vi "Camera.v5.vi"() -> ()   [LabVIEW 2015]
uses:
  Camera Properties.ctl
  Microscope Settings.ctl
  CameraState.ctl
  ModeEnum.ctl
  Stack_State.ctl
  Stack Track.ctl
  CameraControlTypeDef.ctl
  <vilib>/DAQmx/write.llb/DAQmx Write (Analog 1D Wfm NChan NSamp).vi
  <vilib>/DAQmx/create/channels.llb/DAQmx Create Channel (AO-Voltage-Basic).vi
  <vilib>/Waveform/WDTOps.llb/WDT Number of Waveform Samples DBL.vi
  <vilib>/DAQmx/configure/timing.llb/DAQmx Timing (Sample Clock).vi
  <vilib>/DAQmx/miscellaneous.llb/DAQmx Fill In Error Info.vi
  <vilib>/vision/NI_Vision_Development_Module.lvlib
  <vilib>/DAQmx/write.llb/DAQmx Write (Digital 1D Wfm NChan NSamp).vi
panel:
  out "Relax/ms":dbl
  in  "Tab Control":enum32{"Camera Settings", "Recording"}(tab)
  in  "Microscope Settings":T1={"Mode"=enum."XY", {"Scanning Mode"=12.0, "Slit Width /%"=5.0}, "Piezo Position /um"=0.0, "Exposure/ms"=40.0, "Samples per millisecond"=100.0, "Relax/ms"=10.0, "Readout Direction"=2.0, "Trigger Source"=2.0} {"Trigger Source" items=["Internal"=1.0, "External"=2.0]; "Readout Direction" items=["Forward"=1.0, "Backward"=2.0]; "?"."Scanning Mode" items=["Full Frame"=1.0, "Slit Scanning"=12.0]}
  in  "Scan":bool
  in  "Scan Continuously":bool
  out "error IO":errorcluster
  in  "V Height":dbl=2048.0 min=4.0 max=2048.0 step=4.0
  in  "V Offset":dbl min=0.0 max=0.0 step=4.0
  in  "H Offset":dbl min=0.0 max=0.0 step=4.0
  in  "H Width":dbl min=4.0 max=2048.0 step=4.0
  in  "Advanced DCAM Controls":i32(listbox) caption="Multicolumn Listbox"
  in  "Properties":T2=4211904 items=["SENSOR MODE"=4212128, "CCD MODE"=4212384, "READOUT MODE"=4211872, "ACTIVE VIEW INDEX"=4343136, "BITS PER CHANNEL"=4342976, "IMAGE PIXEL TYPE"=4343296, "BINNING"=4215968, "EXPOSURE TIME"=2049184, "CONTRAST GAIN"=3163312, "CONTRAST OFFSET"=3163328, "LIGHT MODE"=2114720, "SENSITIVITY"=2114992, "PHOTON IMAGING MODE"=2115200, "HIGH DYNAMIC RANGE MODE"=3163360, "WHITE BALANCE"=3163568, "TEMPERATURE"=2115232, "TEMPERATURE TARGET"=2115264, "SENSOR COOLER FAN"=2115296, "LINEBUNDLE HEIGHT"=4212192, "MECHANICAL SHUTTER"=2115488, "BACK FOCUS POSITION"=8422304, "TRIGGER CONNECTOR"=1066432, "TRIGGER SOURCE"=1066144, "OUTPUT TRIGGER SOURCE"=1852576, "TRIGGER GLOBAL EXPOSURE"=2049680, "FIRST TRIGGER BEHAVIOR"=2049696, "CHANNEL SYNC"=1852352, "READOUT DIRECTION"=4211904, "PRE HSYNC COUNT"=1852704, "INTERNAL LINE SPEED"=4191408, "INTERNAL LINE INVERVAL"=4191424]
  out "Waves":waveform(dbl)[](graph)
  out "Image":T3(plugin-control)
  out "Histogram":T4(graph)
  in  "stop":bool
  in  "Calibration":bool
  in  "MultiD Scan":bool
  in  "Stage Controller":bool
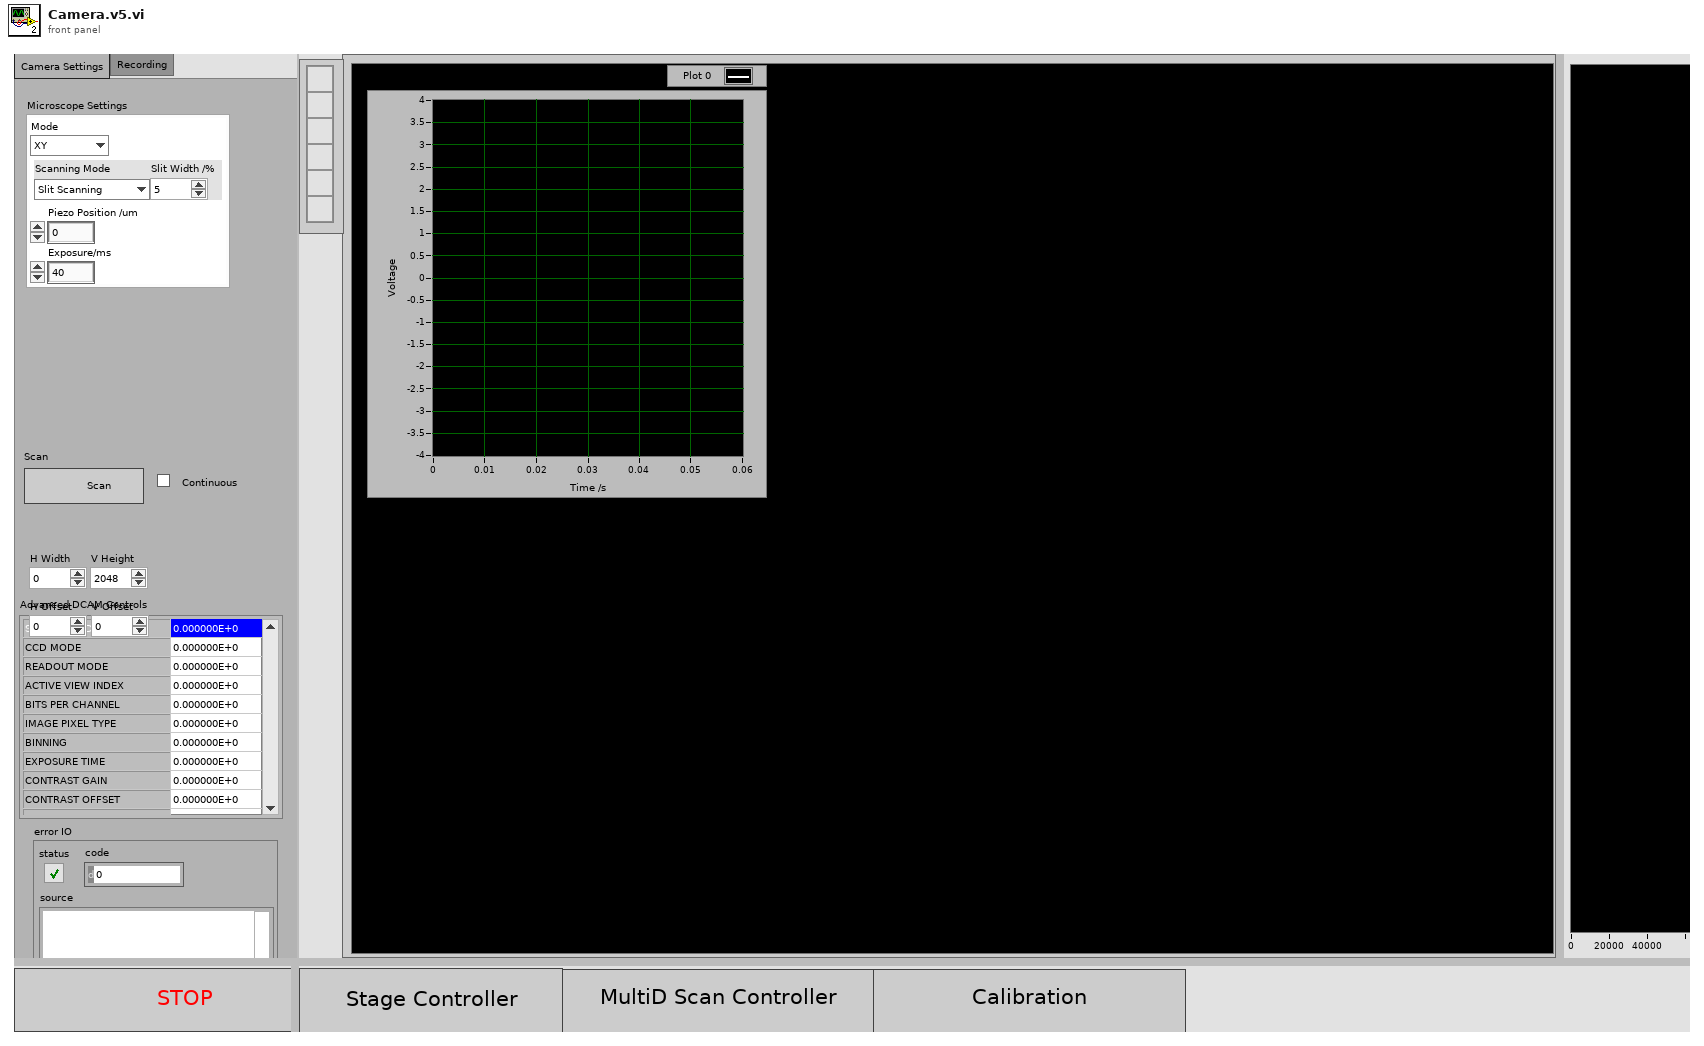
[diagram p1: front panel]
types:
  T1 = typedef "Microscope Settings.ctl" = cluster{"Mode":enum16{"X", "XY", "XYZ", "XYZT", "XYZC"}, cluster{"Scanning Mode":dbl, "Slit Width /%":dbl}, "Piezo Position /um":dbl, "Exposure/ms":dbl, "Samples per millisecond":dbl, "Relax/ms":dbl, "Readout Direction":dbl, "Trigger Source":dbl}
  T2 = typedef "Camera Properties.ctl" = u32
  T3 = typedef "IMAQ Image.ctl" = refnum<image>
  T4 = cluster{"Starting Value":sgl, "Incremental Value":sgl, "Histogram":u32[]}
  T5 = typedef "ModeEnum.ctl" = enum16{"Idle", "generateWaves", "runWaves", "stop"}
  T6 = cluster{"height":u32, "width":u32, "datatype":u32}
  T7 = typedef "CameraState.ctl" = enum16{"init", "active", "deinit"}
  T8 = typedef "CameraControlTypeDef.ctl" = enum16{"IntervalLineInt", "Ram Record", "HardDisk Record", "Disengage Update", "Update", "Idle", "ROI", "Binning", "Scan Mode", "Trigger Mode", "Readout Mode", "Readout Direction", "Preview", "ROIWindow", "Trigger Source"}
  T9 = typedef "Stack_State.ctl" = cluster{"State":T10, "Stack Number":i32, "Image":u16[][], "Stacks":i32}
  T10 = typedef "Stack Track.ctl" = enum16{"Idle", "Display", "Start Sequence", "Read Disk", "STOP", "Collecting", "End"}
  T11 = typedef "Image Type" = u32
  T12 = cluster{"Value":i32, "Minimum":i32, "Maximum":i32, "Increment":i32}
  T13 = cluster{"Minimum":i32, "Maximum":i32, "Increment":i32}
  T14 = cluster{"State":T10, "Timeout":i32, "Data 16":u16[][], "Timeout":i32}
  T15 = cluster{"Enum":T8, "Trigger Source":dbl, "timeout in ms (-1)":i32}
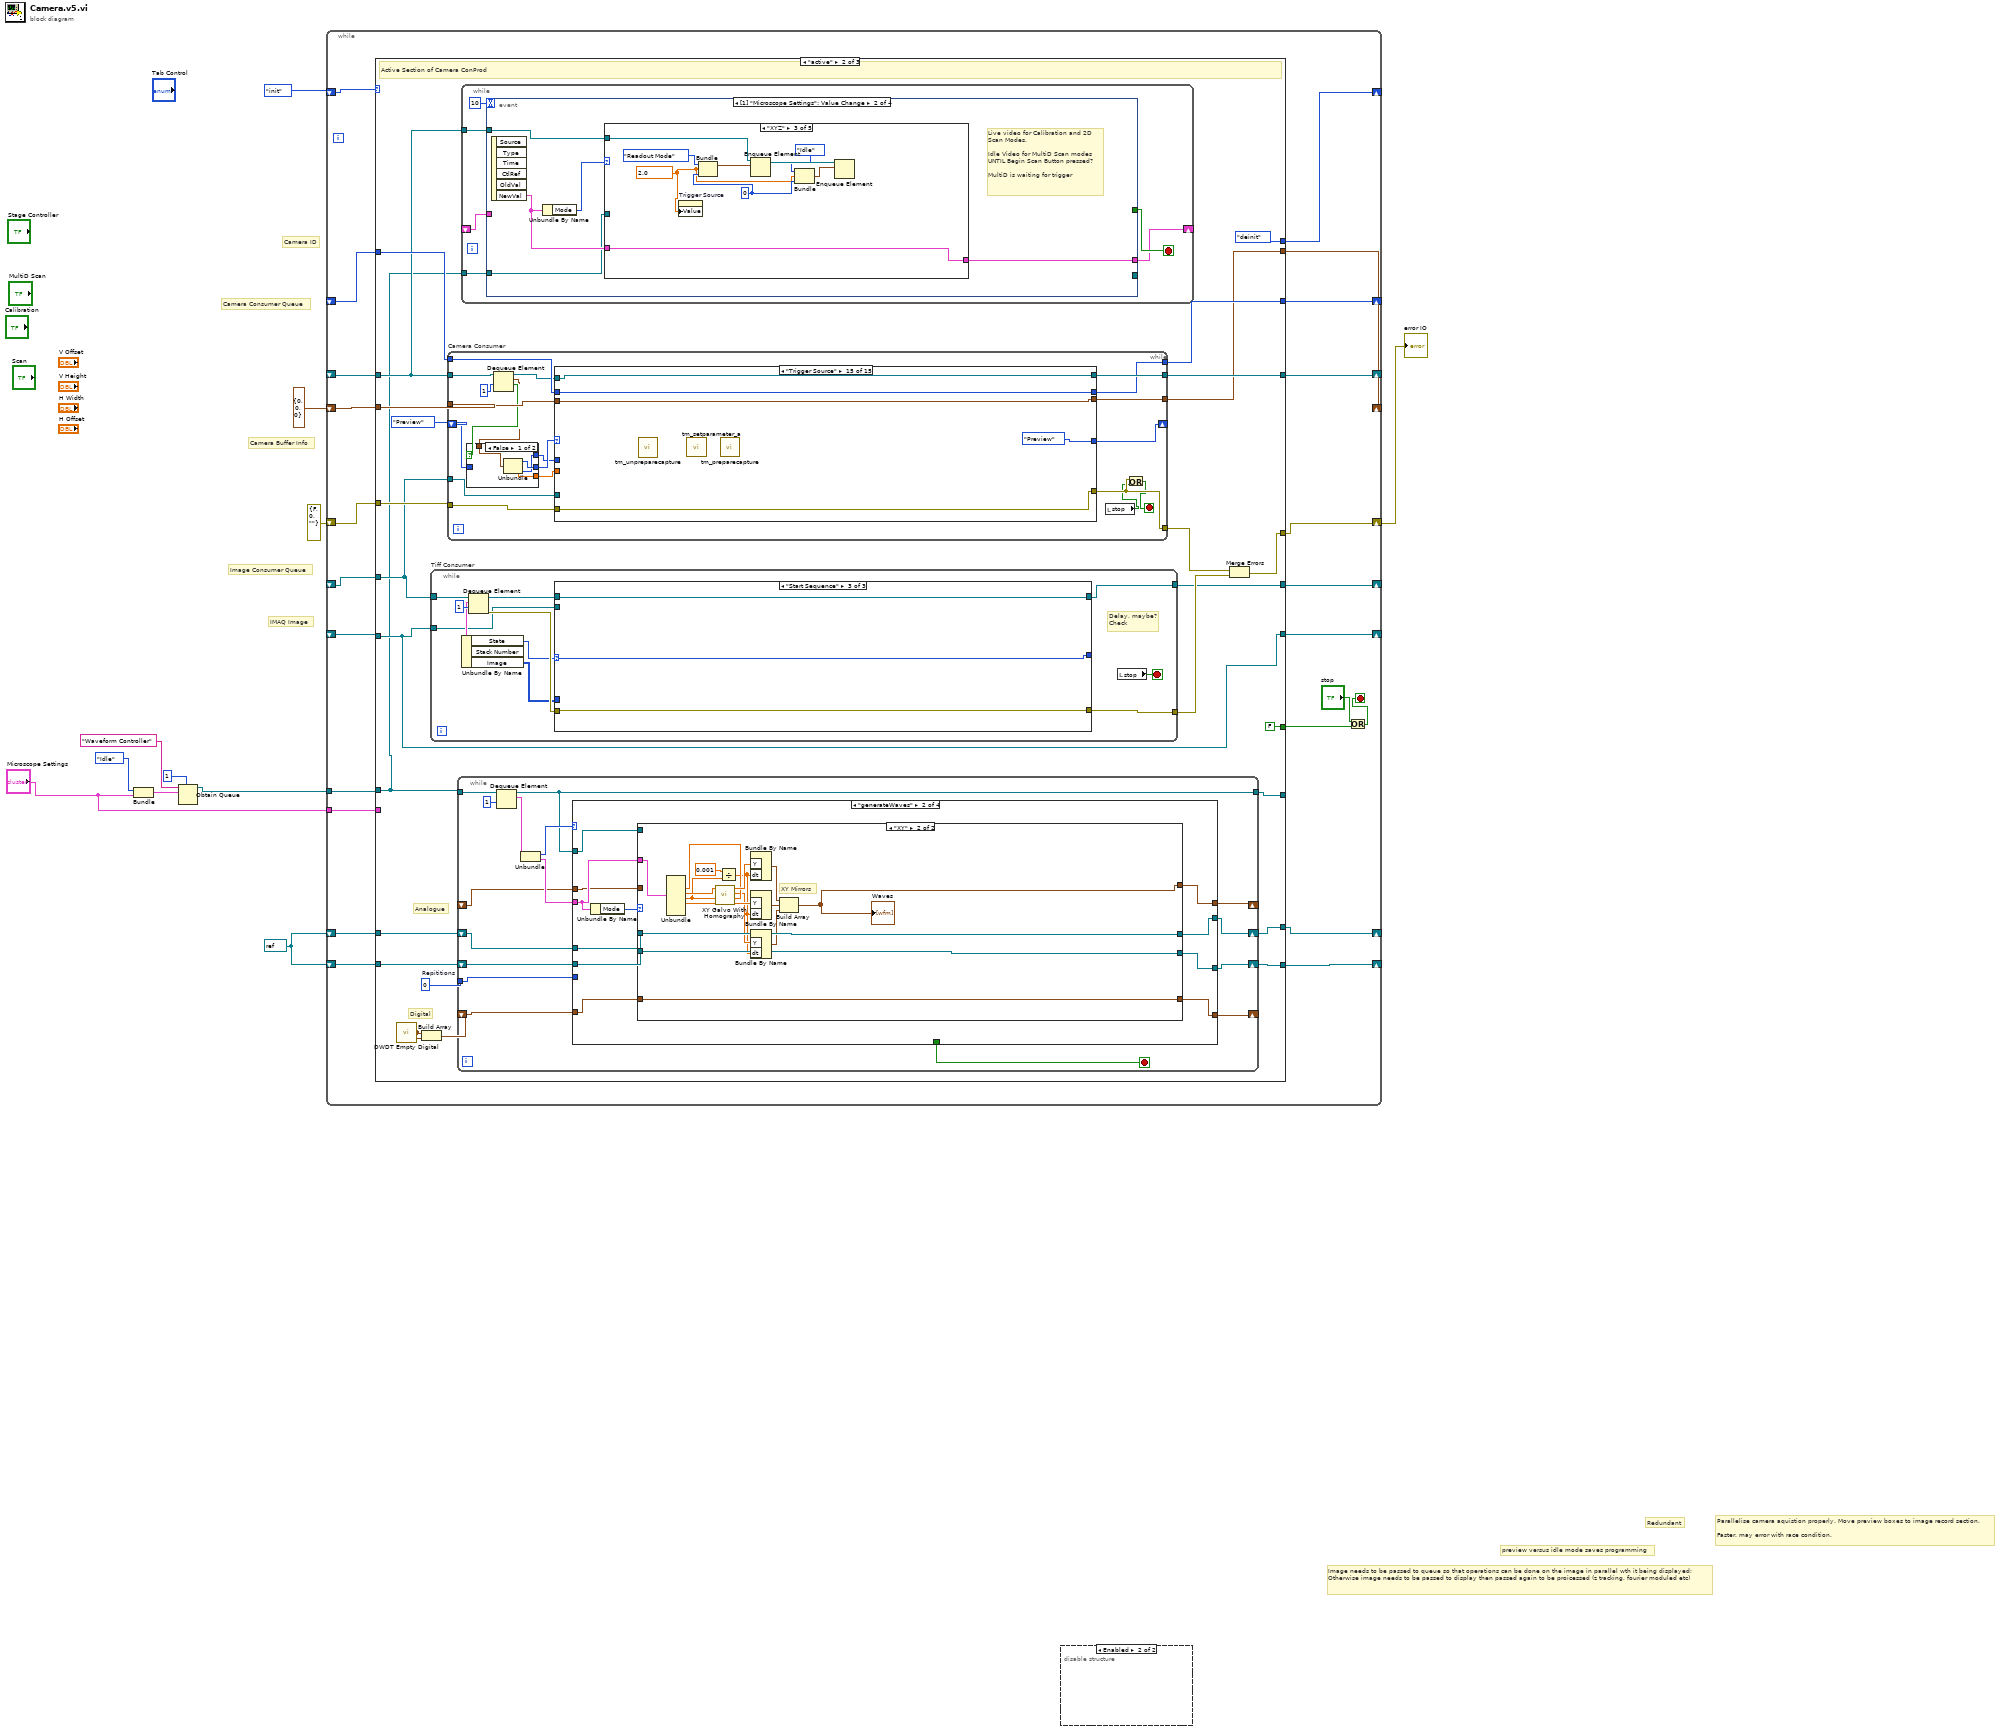
[diagram p0: block diagram]
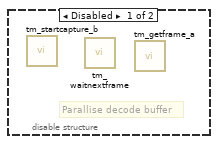
[diagram p2: hidden frame]
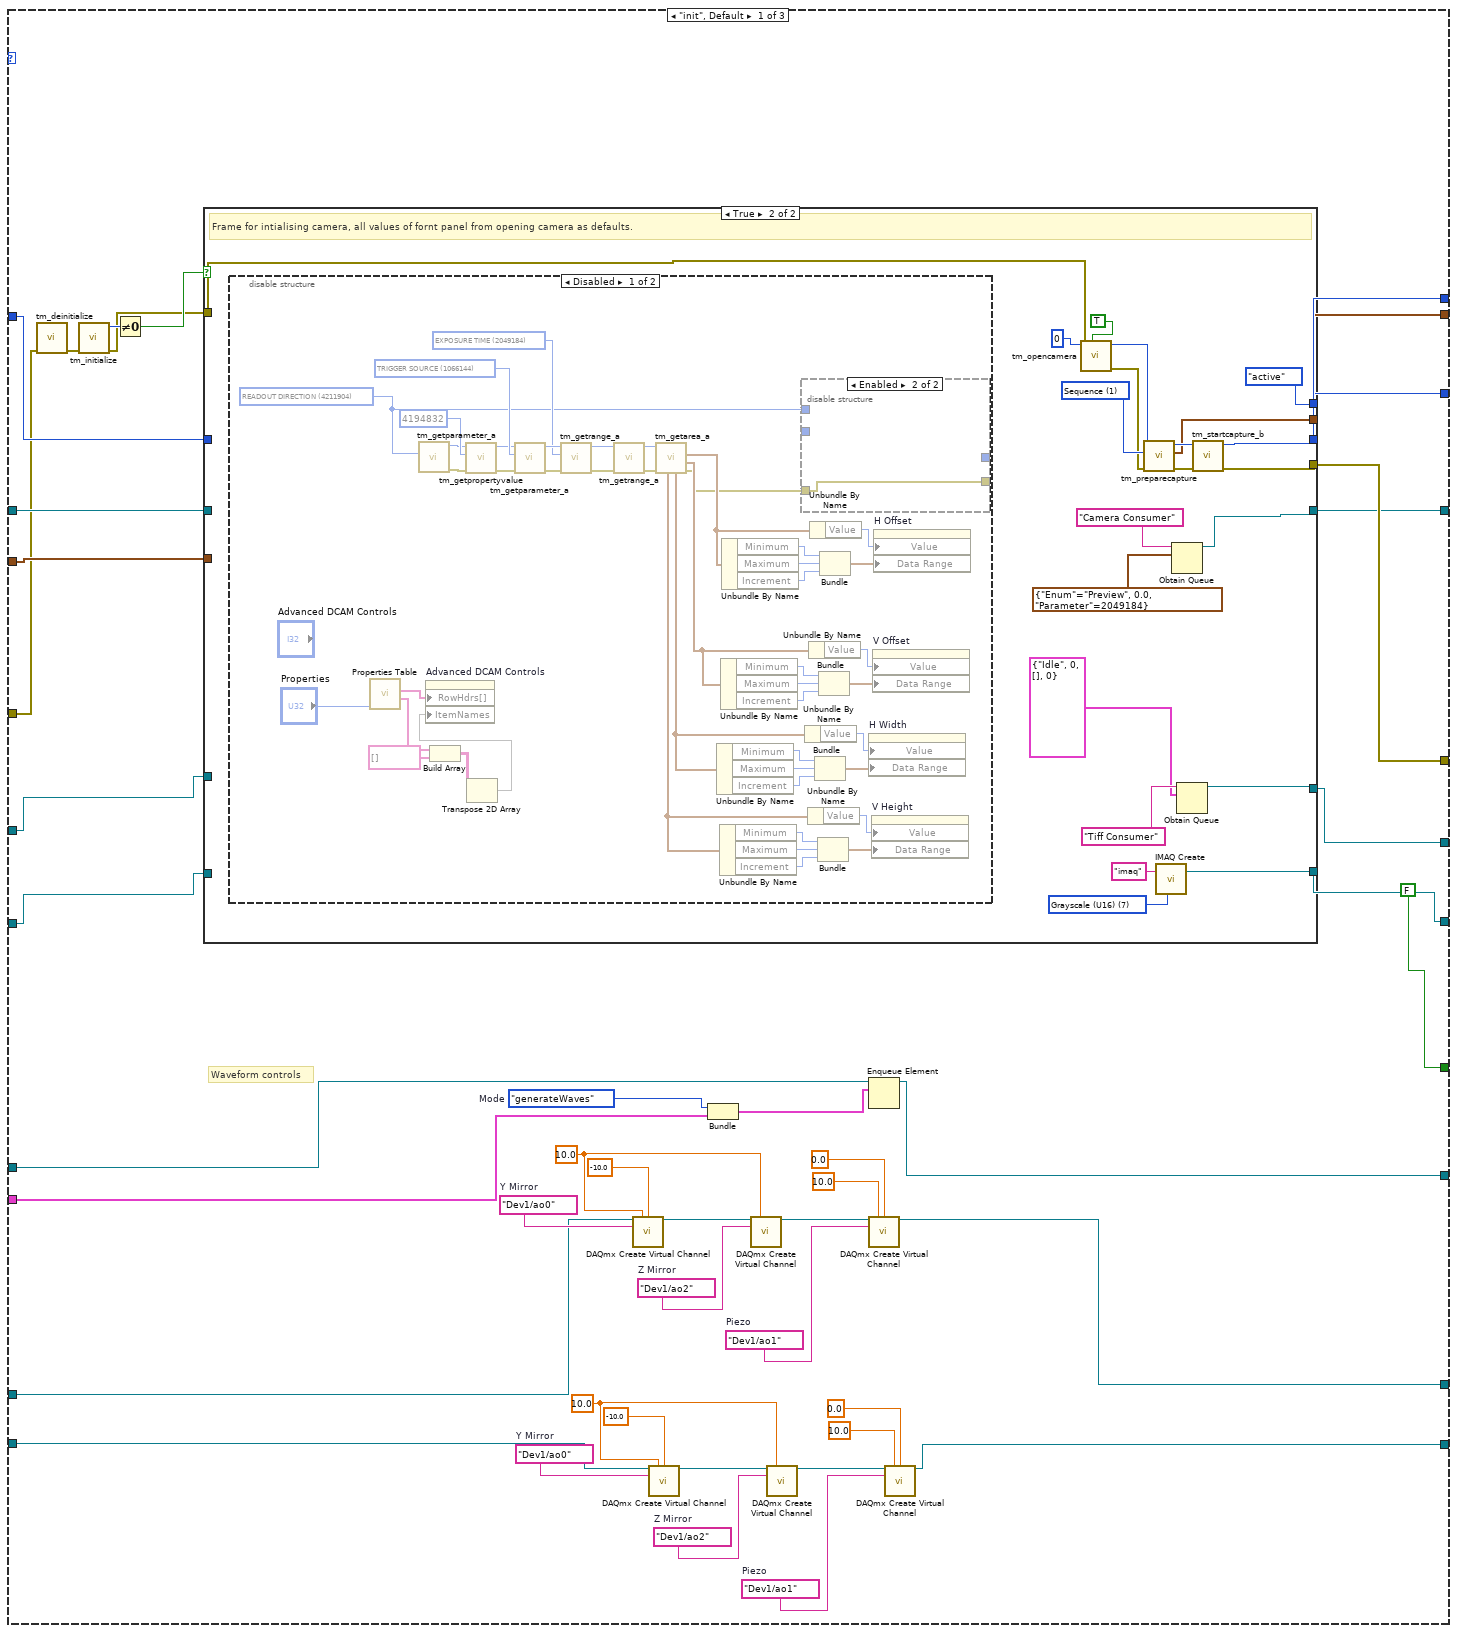
[diagram p3: hidden frame]
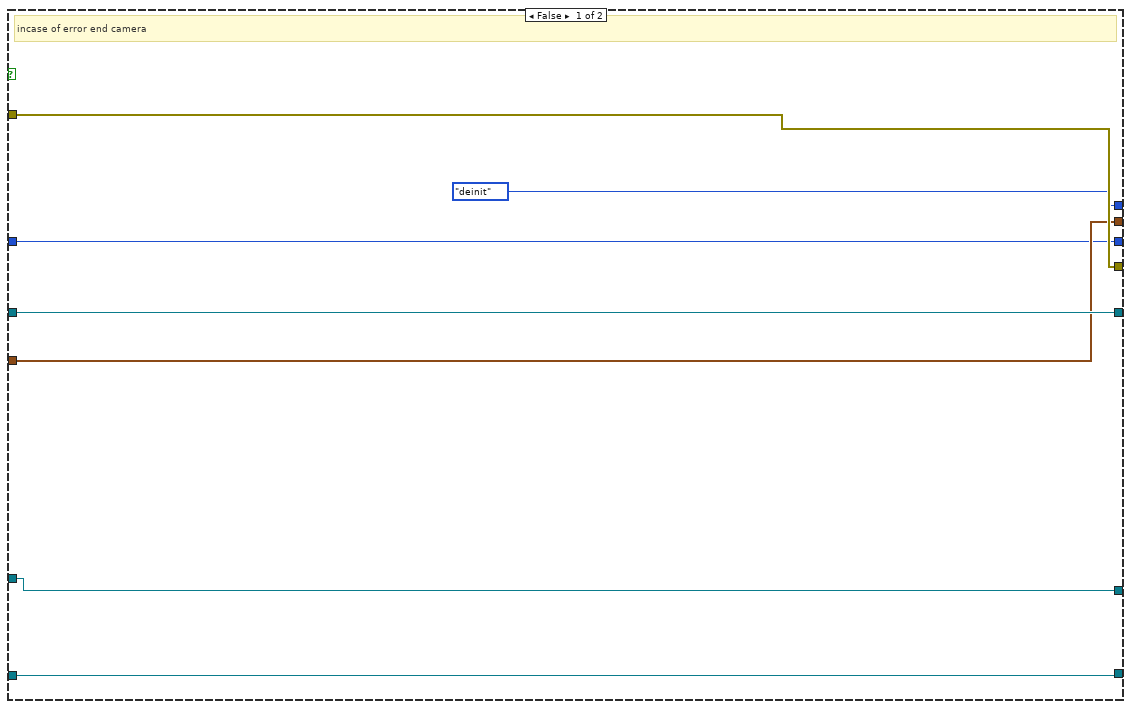
[diagram p4: hidden frame]
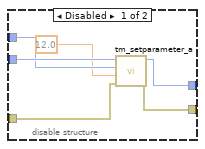
[diagram p5: hidden frame]
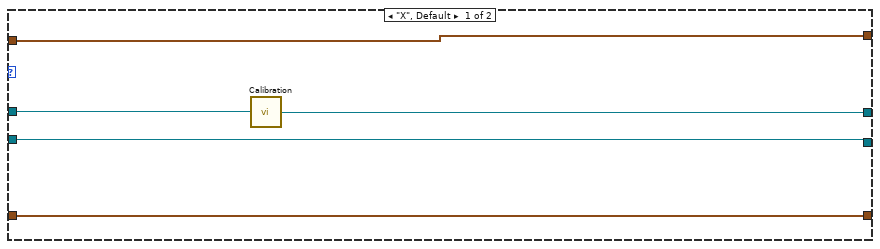
[diagram p8: hidden frame]
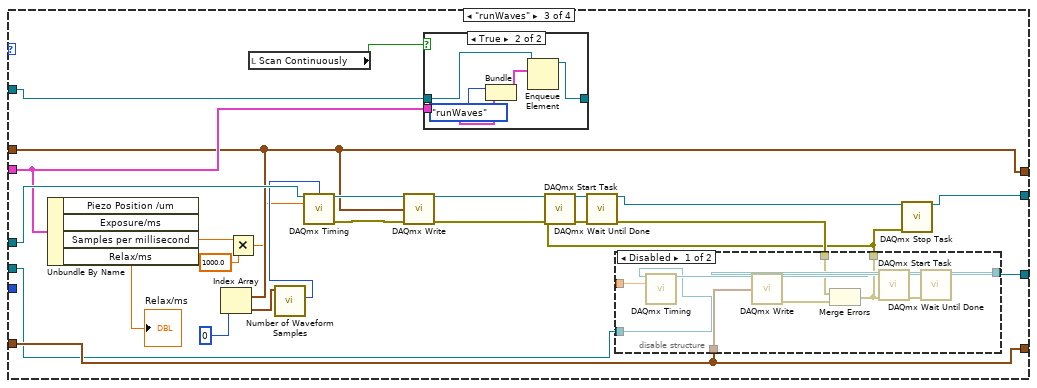
[diagram p9: hidden frame]
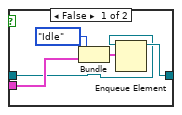
[diagram p11: hidden frame]
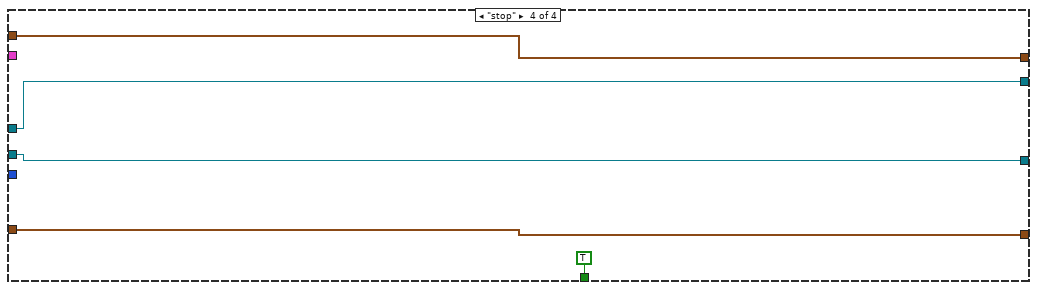
[diagram p12: hidden frame]
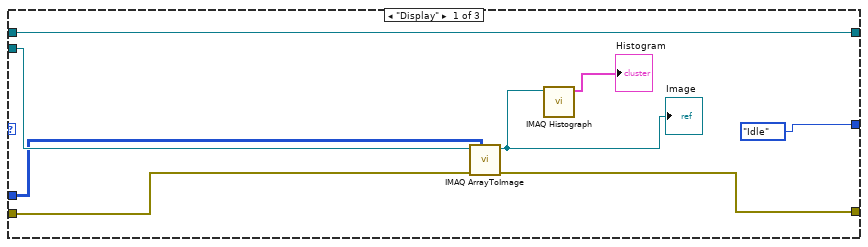
[diagram p13: hidden frame]
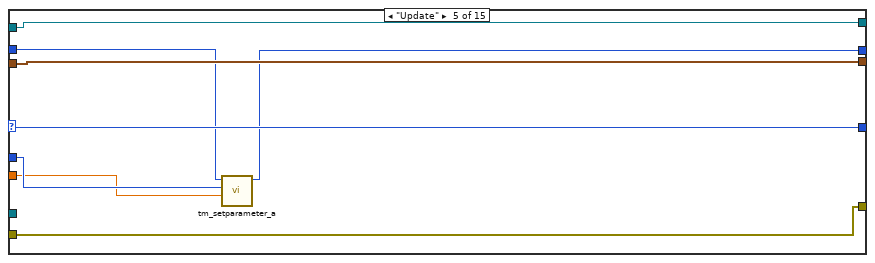
[diagram p20: hidden frame]
diagram:
  w8 = refnum<k21> refnum ("Mirror Z 2")
  # "IMAQ Image"
  # "Camera Buffer Info"
  # "Image needs to be passed to queue so that operations can be done on the image in parallel wth it being displayed;\nOtherwise image needs to be passed to display then passed again to be proicessed (z tracking, fourier moduled etc)"
  # "preview versus idle mode saves programming"
  # "Parallelise camera aquistion properly. Move preview boxes to image record section.\n\nFaster. may error with race condition."
  # "Redundant"
  # "Image Consumer Queue"
  # "Camera Consumer Queue"
  # "Camera ID"
  n1 = Bundle("Mode"=ModeEnum."Idle", "Microscope Settings"="Microscope Settings") -> (w5:cluster{"Mode":T5, "Microscope Settings":T1})  [unwired: 1 in]
  n2 = Obtain Queue(max queue size (-1, unlimited)=1, name (unnamed)="Waveform Controller", element data type=w5) -> (queue out=w1:refnum<queue>)  [unwired: 2 in, 2 out]
  n3 = while {
    shift-right: [w34] -> _
    shift-left: CameraState."init" -> [w33]
    shift-right: [w32] -> _
    shift-left: _ -> [w31]
    shift-right: [w30] -> w10
    shift-left: errorcluster {"status"=FALSE, "code"=0, "source"=""} ("error IO") -> [w29]
    shift-right: [w27] -> _
    shift-left: _ -> [w26]
    shift-right: [w28] -> _
    shift-left: _ -> [w25]
    shift-right: [w21] -> _
    shift-left: T6 {"height"=0, "width"=0, "datatype"=0} ("Buffer Info") -> [w20]
    shift-right: [w19] -> _
    shift-left: _ -> [w18]
    shift-right: [w17] -> _
    shift-left: w8 -> [w16]
    shift-right: [w14] -> _
    shift-left: w8 -> [w15]
    tunnel: "Microscope Settings" -> [w13]
    tunnel: w1 -> [w12]
    stop <- w23 stop-if-true
    n4 = case shown="\"active\"" w33 {
      tunnel: [w75 CameraState."deinit" CameraState."init"] -> w34
      tunnel: [w74 w183 w501] -> w32
      tunnel: w31 -> [w52 w184 w501]
      tunnel: [w73 w182 w504] -> w30
      tunnel: w29 -> [w51 w176 w505]
      tunnel: [w72 w179 w488] -> w28
      tunnel: [w71 w178 w484] -> w27
      tunnel: w26 -> [w69 w171 w484]
      tunnel: w25 -> [w70 w169 w488]
      tunnel: [FALSE ("stop") FALSE ("stop") TRUE ("stop")] -> w22
      tunnel: [w67 w174 w498] -> w21
      tunnel: w20 -> [w66 w173 w498]
      tunnel: w18 -> [w64 w170 w497]
      tunnel: [w65 w170 w497] -> w19
      tunnel: w12 -> [w38 w161 w483]
      tunnel: [w56 w162 w495] -> w17
      tunnel: w16 -> [w53 w165 w495]
      tunnel: w15 -> [w41 w164 w493]
      tunnel: [w40 w163 w493] -> w14
      tunnel: [w39 w160 w483] -> _
      tunnel: w13 -> [w37 _ _]
      frame "init", Default {
        w35 = ModeEnum."generateWaves"  # Mode
        w46 = tag "Dev1/ao1"  # Piezo
        w47 = tag "Dev1/ao2"  # Z Mirror
        w48 = tag "Dev1/ao0"  # Y Mirror
        w50 = 10.0 ("maximum value")
        w59 = tag "Dev1/ao1"  # Piezo
        w60 = tag "Dev1/ao2"  # Z Mirror
        w61 = tag "Dev1/ao0"  # Y Mirror
        w63 = 10.0 ("maximum value")
        # "Waveform controls"
        n5 = call "tm_deinitialize.vi"("error in (no error)"=w51) -> ("error out"=w79:errorcluster)  [unwired: 10 in]
        n6 = call "tm_initialize.vi"("error in (no error)"=w79) -> ("error out"=w76:errorcluster, "Number Of Cameras"=w78:u32)  [unwired: 7 in, 2 out]
        n7 = Not Equal To 0?(x=w78) -> (x != 0?=w77:bool)
        n8 = case shown="True" w77 {
          tunnel: w76 -> [w86 w105]
          tunnel: [CameraState."deinit" CameraState."active"] -> w75
          tunnel: [w86 w102] -> w73
          tunnel: [w81 w100] -> w74
          tunnel: [w84 w87] -> w72
          tunnel: [w83 w97] -> w71
          tunnel: w70 -> [w84 _]
          tunnel: w69 -> [w83 _]
          tunnel: [w82 w95] -> w67
          tunnel: w66 -> [w82 _]
          tunnel: w52 -> [w81 _]
          tunnel: [w80 w92] -> w65
          tunnel: w64 -> [w80 _]
          frame False {
            # "incase of error end camera"
          }
          frame True {
            w94 = T11 7 items=["Grayscale (U8)", "Grayscale (I16)", "Grayscale (SGL)", "Complex (CSG)", "RGB (U32)", "HSL (U32)", "RGB (U64)", "Grayscale (U16)"] ("Image Type")
            w104 = 1 items=["Snap", "Sequence"] ("Capture mode")
            # "Frame for intialising camera, all values of fornt panel from opening camera as defaults."
            n9 = disable-structure shown="Disabled" {
              frame Disabled {
                w149 = u32 2049184 items=["SENSOR MODE"=4212128, "CCD MODE"=4212384, "READOUT MODE"=4211872, "ACTIVE VIEW INDEX"=4343136, "BITS PER CHANNEL"=4342976, "IMAGE PIXEL TYPE"=4343296, "BINNING"=4215968, "EXPOSURE TIME"=2049184, "CONTRAST GAIN"=3163312, "CONTRAST OFFSET"=3163328, "LIGHT MODE"=2114720, "SENSITIVITY"=2114992, "PHOTON IMAGING MODE"=2115200, "HIGH DYNAMIC RANGE MODE"=3163360, "WHITE BALANCE"=3163568, "TEMPERATURE"=2115232, "TEMPERATURE TARGET"=2115264, "SENSOR COOLER FAN"=2115296, "LINEBUNDLE HEIGHT"=4212192, "MECHANICAL SHUTTER"=2115488, "BACK FOCUS POSITION"=8422304, "TRIGGER CONNECTOR"=1066432, "TRIGGER SOURCE"=1066144, "OUTPUT TRIGGER SOURCE"=1852576, "TRIGGER GLOBAL EXPOSURE"=2049680, "FIRST TRIGGER BEHAVIOR"=2049696, "CHANNEL SYNC"=1852352, "READOUT DIRECTION"=4211904, "PRE HSYNC COUNT"=1852704, "INTERNAL LINE SPEED"=4191408, "INTERNAL LINE INVERVAL"=4191424] ("Parameter")
                w109 = T2 4211904 items=["SENSOR MODE"=4212128, "CCD MODE"=4212384, "READOUT MODE"=4211872, "ACTIVE VIEW INDEX"=4343136, "BITS PER CHANNEL"=4342976, "IMAGE PIXEL TYPE"=4343296, "BINNING"=4215968, "EXPOSURE TIME"=2049184, "CONTRAST GAIN"=3163312, "CONTRAST OFFSET"=3163328, "LIGHT MODE"=2114720, "SENSITIVITY"=2114992, "PHOTON IMAGING MODE"=2115200, "HIGH DYNAMIC RANGE MODE"=3163360, "WHITE BALANCE"=3163568, "TEMPERATURE"=2115232, "TEMPERATURE TARGET"=2115264, "SENSOR COOLER FAN"=2115296, "LINEBUNDLE HEIGHT"=4212192, "MECHANICAL SHUTTER"=2115488, "BACK FOCUS POSITION"=8422304, "TRIGGER CONNECTOR"=1066432, "TRIGGER SOURCE"=1066144, "OUTPUT TRIGGER SOURCE"=1852576, "TRIGGER GLOBAL EXPOSURE"=2049680, "FIRST TRIGGER BEHAVIOR"=2049696, "CHANNEL SYNC"=1852352, "READOUT DIRECTION"=4211904, "PRE HSYNC COUNT"=1852704, "INTERNAL LINE SPEED"=4191408, "INTERNAL LINE INVERVAL"=4191424] ("Parameter")
                w152 = u32 1066144 items=["SENSOR MODE"=4212128, "CCD MODE"=4212384, "READOUT MODE"=4211872, "ACTIVE VIEW INDEX"=4343136, "BITS PER CHANNEL"=4342976, "IMAGE PIXEL TYPE"=4343296, "BINNING"=4215968, "EXPOSURE TIME"=2049184, "CONTRAST GAIN"=3163312, "CONTRAST OFFSET"=3163328, "LIGHT MODE"=2114720, "SENSITIVITY"=2114992, "PHOTON IMAGING MODE"=2115200, "HIGH DYNAMIC RANGE MODE"=3163360, "WHITE BALANCE"=3163568, "TEMPERATURE"=2115232, "TEMPERATURE TARGET"=2115264, "SENSOR COOLER FAN"=2115296, "LINEBUNDLE HEIGHT"=4212192, "MECHANICAL SHUTTER"=2115488, "BACK FOCUS POSITION"=8422304, "TRIGGER CONNECTOR"=1066432, "TRIGGER SOURCE"=1066144, "OUTPUT TRIGGER SOURCE"=1852576, "TRIGGER GLOBAL EXPOSURE"=2049680, "FIRST TRIGGER BEHAVIOR"=2049696, "CHANNEL SYNC"=1852352, "READOUT DIRECTION"=4211904, "PRE HSYNC COUNT"=1852704, "INTERNAL LINE SPEED"=4191408, "INTERNAL LINE INVERVAL"=4191424] ("Parameter")
                n10 = call "Properties Table.vi"("Properties"="Properties") -> ("Value Stirngs Out"=w114:string[], "Row Headers"=w115:string[])  [unwired: 4 in, 2 out]
                n11 = call "tm_getparameter_a.vi"("Parameter"=w109) -> ("error out"=w141:errorcluster, "Handle out"=w143:u32)  [unwired: 8 in, 1 out]
                n12 = Build Array(w114, string[] [] ("element")) -> (w112:string[][])
                n13 = call "tm_getpropertyvalue.vi"("error in (no error)"=w141, "Property ID"=u32 4194832, "Handle in"=w143) -> ("error out"=w142:errorcluster, "Handle out"=w108:u32)  [unwired: 6 in, 1 out]
                n14 = Transpose 2D Array(2D array=w112) -> (transposed array=w111:string[][])
                n15 = property on="Advanced DCAM Controls" class="MCListbox (strict)"("RowHdrs[]"=w115, "ItemNames"=w111) -> ()  [unwired: 2 in, 2 out]
                n16 = call "tm_getparameter_a.vi"("error in (no error)"=w142, "Parameter"=w152, "Handle in"=w108) -> ("error out"=w150:errorcluster, "Handle out"=w151:u32)  [unwired: 6 in, 1 out]
                n17 = call "tm_getrange_a.vi"("error in (no error)"=w150, "Parameter"=w149, "Handle in"=w151) -> ("error out"=w147:errorcluster, "Handle out"=w148:u32)  [unwired: 2 in, 5 out]
                n18 = call "tm_getrange_a.vi"("error in (no error)"=w147, "Handle in"=w148) -> ("error out"=w146:errorcluster, "Handle out"=w145:u32)  [unwired: 3 in, 5 out]
                n19 = call "tm_getarea_a.vi"("error in (no error)"=w146, "Handle in"=w145) -> ("error out"=w110:errorcluster, "V Offset"=w117:T12, "H Offset"=w140:T12, "H Width"=w118:T12, "V Width"=w119:T12)  [unwired: 4 in, 1 out]
                n20 = Unbundle By Name(w118) -> ("Minimum"=w129:i32, "Maximum"=w128:i32, "Increment"=w127:i32)
                n21 = Unbundle By Name(w119) -> ("Minimum"=w120:i32, "Maximum"=w121:i32, "Increment"=w122:i32)
                n22 = Unbundle By Name(w117) -> ("Minimum"=w130:i32, "Maximum"=w131:i32, "Increment"=w132:i32)
                n23 = Unbundle By Name(w140) -> ("Minimum"=w139:i32, "Maximum"=w138:i32, "Increment"=w137:i32)
                n24 = disable-structure shown="Enabled" {
                  disable-tunnel: _ -> [w158 _]
                  disable-tunnel: [w157 _] -> _
                  disable-tunnel: w110 -> [w156 w159]
                  disable-tunnel: [w155 w159] -> _
                  disable-tunnel: w109 -> [w154 _]
                  frame Disabled {
                    n25 = call "tm_setparameter_a.vi"("error in (no error)"=w156, "Value in"=12.0, "Parameter"=w154, "Handle in"=w158) -> ("error out"=w155:errorcluster, "Handle out"=w157:u32)  [unwired: 6 in]
                  }
                  frame Enabled {
                  }
                }
                n26 = Unbundle By Name(w118) -> ("Value"=w125:i32)
                n27 = Unbundle By Name(w119) -> ("Value"=w124:i32)
                n28 = Unbundle By Name(w117) -> ("Value"=w134:i32)
                n29 = Unbundle By Name(w140) -> ("Value"=w135:i32)
                n30 = Bundle("Minimum"=w129, "Maximum"=w128, "Increment"=w127) -> (w126:T13)  [unwired: 1 in]
                n31 = Bundle("Minimum"=w120, "Maximum"=w121, "Increment"=w122) -> (w123:T13)  [unwired: 1 in]
                n32 = Bundle("Minimum"=w130, "Maximum"=w131, "Increment"=w132) -> (w133:T13)  [unwired: 1 in]
                n33 = Bundle("Minimum"=w139, "Maximum"=w138, "Increment"=w137) -> (w136:T13)  [unwired: 1 in]
                n34 = property on="H Width" class="DigNum (strict)"("Value"=w125, "Data Range"=w126) -> ()  [unwired: 2 in, 2 out]
                n35 = property on="V Height" class="DigNum (strict)"("Value"=w124, "Data Range"=w123) -> ()  [unwired: 2 in, 2 out]
                n36 = property on="V Offset" class="DigNum (strict)"("Value"=w134, "Data Range"=w133) -> ()  [unwired: 2 in, 2 out]
                n37 = property on="H Offset" class="DigNum (strict)"("Value"=w135, "Data Range"=w136) -> ()  [unwired: 2 in, 2 out]
              }
              frame Enabled {
              }
            }
            n38 = call "tm_opencamera.vi"("Force Open"=TRUE, "error in (no error)"=w105, "Camera Index"=u32 0) -> ("error out"=w89:errorcluster, "Handle out"=w88:u32)  [unwired: 6 in, 1 out]
            n39 = call "tm_preparecapture.vi"("error in (no error)"=w89, "Capture mode"=w104, "Handle in"=w88) -> ("error out"=w103:errorcluster, "Buffer Info"=w95:T6, "Handle out"=w101:u32)  [unwired: 5 in, 1 out]
            n40 = call "IMAQ Create"("Image Name"="imaq", "Image Type"=w94) -> ("New Image"=w92:T3)  [unwired: 3 in, 1 out]
            n41 = Obtain Queue(name (unnamed)="Camera Consumer", element data type=cluster{"Enum":T8, dbl, "Parameter":u32} {"Enum"=enum."Preview", 0.0, "Parameter"=2049184}) -> (queue out=w87:refnum<queue>)  [unwired: 3 in, 2 out]
            n42 = Obtain Queue(name (unnamed)="Tiff Consumer", element data type=T9 {"State"=enum."Idle", "Stack Number"=0, "Image"=[], "Stacks"=0} ("input cluster")) -> (queue out=w97:refnum<queue>)  [unwired: 3 in, 2 out]
            n43 = call "tm_startcapture_b.vi"("error in (no error)"=w103, "Handle in"=w101) -> ("error out"=w102:errorcluster, "Handle out"=w100:u32)  [unwired: 8 in]
          }
        }
        n44 = call-poly <vilib>:"DAQmx Create Virtual Channel.vi"("task in"=w53, "maximum value"=w63, "minimum value"=-10.0, "physical channels"=w61) -> ("task out"=w55:refnum<k21>)  [unwired: 10 in, 1 out]
        n45 = call-poly <vilib>:"DAQmx Create Virtual Channel.vi"("task in"=w41, "maximum value"=w50, "minimum value"=-10.0, "physical channels"=w48) -> ("task out"=w43:refnum<k21>)  [unwired: 10 in, 1 out]
        n46 = Bundle("Mode"=w35, "Microscope Settings"=w37) -> (w36:cluster{"Mode":T5, "Microscope Settings":T1})  [unwired: 1 in]
        n47 = call-poly <vilib>:"DAQmx Create Virtual Channel.vi"("task in"=w55, "maximum value"=w63, "physical channels"=w60) -> ("task out"=w54:refnum<k21>)  [unwired: 11 in, 1 out]
        n48 = call-poly <vilib>:"DAQmx Create Virtual Channel.vi"("task in"=w43, "maximum value"=w50, "physical channels"=w47) -> ("task out"=w42:refnum<k21>)  [unwired: 11 in, 1 out]
        n49 = Enqueue Element(queue=w38, element=w36) -> (queue out=w39:refnum<queue>)  [unwired: 2 in, 2 out]
        n50 = call-poly <vilib>:"DAQmx Create Virtual Channel.vi"("task in"=w54, "maximum value"=10.0 ("minimum value"), "minimum value"=0.0 ("maximum value"), "physical channels"=w59) -> ("task out"=w56:refnum<k21>)  [unwired: 10 in, 1 out]
        n51 = call-poly <vilib>:"DAQmx Create Virtual Channel.vi"("task in"=w42, "maximum value"=10.0 ("minimum value"), "minimum value"=0.0 ("maximum value"), "physical channels"=w46) -> ("task out"=w40:refnum<k21>)  [unwired: 10 in, 1 out]
      }
      frame "active" {
        w168 = 0  # Repititions
        # "Digital"
        # "Analogue"
        # "Active Section of Camera ConProd"
        n52 = call <vilib>:"DWDT Empty Digital.vi"() -> ("digital waveform out"=w166:digitalwaveform)  [unwired: 5 in]
        n53 = Build Array(w166, w166) -> (w167:digitalwaveform[])
        n54 = while "Tiff Consumer" {
          tunnel: [w293] -> w181
          tunnel: [w296] -> w178
          tunnel: w171 -> [w298]
          tunnel: w170 -> [w290]
          stop <- w300 stop-if-true
          # "Delay, maybe?\nCheck"
          n55 = Dequeue Element(queue=w298, timeout in ms (-1)=1) -> (queue out=w295:refnum<queue>, element=w297:T9, error out=w294:errorcluster)  [unwired: 1 in, 1 out]
          n56 = Unbundle By Name(w297) -> ("State"=w291:T10, "Image"=w292:u16[][])  [unwired: 1 out]
          n57 = case shown="\"Start Sequence\"" w291 {
            selector: w291 -> [_ w311 w312]
            tunnel: [w308 w310 w313] -> w296
            tunnel: w295 -> [w308 w310 w313]
            tunnel: [Stack_Track."Idle" ("State") w311 w312] -> _
            tunnel: w292 -> [w303 _ _]
            tunnel: w290 -> [w307 _ _]
            tunnel: w294 -> [w306 w309 w314]
            tunnel: [w305 w309 w314] -> w293
            frame "Display" {
              n58 = call "IMAQ ArrayToImage"("Image Pixels (U16)"=w303, "error in (no error)"=w306, "Image"=w307) -> ("error out"=w305:errorcluster, "Image Out"=w302:T3)  [unwired: 7 in]
              "Image" <- w302
              n59 = call "IMAQ Histograph"("Image"=w302) -> ("Histogram Graph"=→"Histogram":T4)  [unwired: 7 in, 3 out]
            }
            frame "Idle", Default {
            }
            frame "Start Sequence" {
            }
          }
          n60 = local read "stop"() -> (w300:bool)
        }
        n61 = while "Camera Consumer" {
          tunnel: w176 -> [w333]
          tunnel: w184 -> [w331]
          tunnel: [w330] -> w183
          tunnel: [w317] -> w180
          tunnel: w169 -> [w326]
          tunnel: [w334] -> w179
          shift-right: [w332] -> _
          shift-left: CameraControlTypeDef."Preview" ("Enum") -> [w322]
          tunnel: [w329] -> w174
          tunnel: w173 -> [w328]
          tunnel: w171 -> [w321]
          stop <- w315 stop-if-true
          n62 = Dequeue Element(queue=w326, timeout in ms (-1)=1) -> (queue out=w325:refnum<queue>, element=w320:cluster{"Enum":T8, dbl, "Parameter":u32}, timed out?=w324:bool)  [unwired: 1 in, 1 out]
          n63 = case shown="False" w324 {
            tunnel: [w337 w339] -> w323
            tunnel: w322 -> [_ w339]
            tunnel: w320 -> [w338 _]
            tunnel: [w336 _] -> w319
            tunnel: [w335 w339] -> w318
            frame False {
              n64 = Unbundle(w338) -> ("Enum"=w337:T8, w336:dbl, "Parameter"=w335:u32)
            }
            frame True {
            }
          }
          n65 = case shown="\"Trigger Source\"" w323 {
            selector: w323 -> [w343 w348 w353 w358 w366 w371 w376 w381 w386 w391 w396 w401 _ w422 _]
            tunnel: w325 -> [w342 w349 w354 w359 w367 w372 w377 w382 w387 w392 w397 w402 w419 w424 w429]
            tunnel: [w342 w349 w354 w359 w367 w372 w377 w382 w387 w392 w397 w402 w419 w424 w429] -> w334
            tunnel: w333 -> [w344 w347 w352 w357 w365 w370 w375 w380 w385 w390 w395 w400 w406 w421 w427]
            tunnel: [w344 w347 w352 w357 w365 w370 w375 w380 w385 w390 w395 w400 w403 w421 w427] -> w317
            tunnel: [w343 w348 w353 w358 w366 w371 w376 w381 w386 w391 w396 w401 CameraControlTypeDef."Preview" ("Enum") w422 CameraControlTypeDef."Preview" ("Enum")] -> w332
            tunnel: w331 -> [w341 w346 w351 w356 w363 w369 w374 w379 w384 w389 w394 w399 w417 w423 w428]
            tunnel: [w341 w346 w351 w356 w362 w369 w374 w379 w384 w389 w394 w399 w415 w423 w428] -> w330
            tunnel: [w340 w345 w350 w355 w364 w368 w373 w378 w383 w388 w393 w398 w412 w420 w426] -> w329
            tunnel: w328 -> [w340 w345 w350 w355 w364 w368 w373 w378 w383 w388 w393 w398 w412 w420 w426]
            tunnel: w321 -> [_ _ _ _ _ _ _ _ _ _ _ _ w411 _ _]
            tunnel: w319 -> [_ _ _ _ w360 _ _ _ _ _ _ _ _ _ _]
            tunnel: w318 -> [_ _ _ _ w361 _ _ _ _ _ _ _ _ _ _]
            frame "IntervalLineInt" {
            }
            frame "Ram Record" {
            }
            frame "HardDisk Record" {
            }
            frame "Disengage Update" {
            }
            frame "Update" {
              n66 = call "tm_setparameter_a.vi"("Value in"=w360, "Parameter"=w361, "Handle in"=w363) -> ("Handle out"=w362:u32)  [unwired: 7 in, 1 out]
            }
            frame "Idle", Default {
            }
            frame "ROI" {
            }
            frame "Binning" {
            }
            frame "Scan Mode" {
            }
            frame "Trigger Mode" {
            }
            frame "Readout Mode" {
            }
            frame "Readout Direction" {
            }
            frame "Preview" {
              w408 = 0 ("Timeout")
              n67 = call "tm_waitnextframe.vi"("error in (no error)"=w406, "Timeout"=3000, "Handle in"=w417) -> ("error out"=w414:errorcluster, "Handle out"=w416:u32)  [unwired: 5 in, 2 out]
              n68 = call "tm_getframe_a.vi"("error in (no error)"=w414, "Buffer Info"=w412, "Handle in"=w416) -> ("error out"=w404:errorcluster, "Data 16"=w409:u16[][], "Handle out"=w415:u32)  [unwired: 4 in, 2 out]
              n69 = Bundle("State"=Stack_Track."Display", "Timeout"=w408, "Data 16"=w409, "Timeout"=w408) -> (w407:T14)  [unwired: 1 in]
              n70 = Enqueue Element(queue=w411, element=w407, error in (no error)=w406) -> (error out=w405:errorcluster)  [unwired: 1 in, 2 out]
              n71 = Merge Errors(w404, w405) -> (w403:errorcluster)
            }
            frame "ROIWindow" {
            }
            frame "Trigger Source" {
              n72 = call "tm_unpreparecapture.vi"() -> ()  [unwired: 10 in, 2 out]
              n73 = call "tm_setparameter_a.vi"() -> ()  [unwired: 10 in, 2 out]
              n74 = call "tm_preparecapture.vi"() -> ()  [unwired: 8 in, 4 out]
            }
          }
          n75 = local read "stop"() -> (w316:bool)
          n76 = Or(x=w317, y=w316) -> (x .or. y?=w315:bool)
        }
        n77 = while {
          tunnel: w161 -> [w200]
          shift-right: [w195] -> _
          shift-left: _ -> [w194]
          tunnel: w168 -> [w193]
          shift-right: [w189] -> w162
          shift-left: w165 -> [w188]
          shift-right: [w192] -> _
          shift-left: w167 -> [w191]
          shift-right: [w187] -> w163
          shift-left: w164 -> [w186]
          tunnel: [w185] -> w160
          stop <- w199 stop-if-true
          n78 = Dequeue Element(queue=w200, timeout in ms (-1)=1) -> (queue out=w185:refnum<queue>, element=w198:cluster{"Mode":T5, "Microscope Settings":T1})  [unwired: 1 in, 2 out]
          n79 = Unbundle(w198) -> ("Mode"=w197:T5, "Microscope Settings"=w196:T1)
          n80 = case shown="\"generateWaves\"" w197 {
            tunnel: [_ _ _ TRUE] -> w199
            tunnel: w196 -> [_ w214 w251 _]
            tunnel: [w204 w215 w249 w289] -> w195
            tunnel: w194 -> [w204 w206 w249 w289]
            tunnel: w193 -> [_ _ _ _]
            tunnel: w185 -> [_ w205 w252 _]
            tunnel: [w201 w210 w256 w288] -> w187
            tunnel: [w202 w208 w243 w287] -> w189
            tunnel: w188 -> [w202 w207 w253 w287]
            tunnel: [w203 w213 w260 w286] -> w192
            tunnel: w191 -> [w203 w212 w260 w286]
            tunnel: w186 -> [w201 w211 w254 w288]
            frame "Idle", Default {
            }
            frame "generateWaves" {
              n81 = Unbundle By Name(w214) -> ("Mode"=w209:enum16{"X", "XY", "XYZ", "XYZT", "XYZC"})
              n82 = case shown="\"XY\"" w209 {
                tunnel: [w220 w224] -> w215
                tunnel: w214 -> [_ w227]
                tunnel: [w218 w230] -> w213
                tunnel: w212 -> [w218 w230]
                tunnel: w211 -> [w219 w229]
                tunnel: [w219 w229] -> w210
                tunnel: [w216 w228] -> w208
                tunnel: w207 -> [w217 w228]
                tunnel: w206 -> [w220 _]
                tunnel: w205 -> [_ _]
                frame "X", Default {
                  n83 = call "Calibration.vi"("Analogue In"=w217) -> ("Analogue In Out"=w216:refnum<k21>)
                }
                frame "XY" {
                  # "XY Mirrors"
                  n84 = Unbundle(w227) -> ("Piezo Position /um"=w233:dbl, "Exposure/ms"=w231:dbl, "Samples per millisecond"=w222:dbl, "Relax/ms"=w232:dbl)  [unwired: 4 out]
                  n85 = call "XY Galvo With Homography.vi"("Piezo Position (um)"=w233, "Relax (ms)"=w232, "Samples /Millisecond"=w222, "Exposure (ms)"=w231) -> ("Z Mirror Signal"=w236:dbl[], "Piezo Signal"=w226:dbl[], "Scan Mirror Signal"=w237:dbl[])  [unwired: 2 in]
                  n86 = Divide(x=0.001 ("y"), y=w222) -> (x/y=w223:dbl)
                  n87 = Bundle By Name("Y"=w237, "dt"=w223) -> (w234:waveform(dbl))  [unwired: 1 in]
                  n88 = Bundle By Name("Y"=w236, "dt"=w223) -> (w235:waveform(dbl))  [unwired: 1 in]
                  n89 = Bundle By Name("Y"=w226, "dt"=w223) -> (w225:waveform(dbl))  [unwired: 1 in]
                  n90 = Build Array(w234, w235, w225) -> (w224:waveform(dbl)[])
                  "Waves" <- w224
                }
              }
            }
            frame "runWaves" {
              n91 = Unbundle By Name(w251) -> ("Samples per millisecond"=w241:dbl, "Relax/ms"=→"Relax/ms":dbl)  [unwired: 2 out]
              n92 = Index Array(array=w249, index=0) -> (element=w247:waveform(dbl))
              n93 = Multiply(x=w241, y=1000.0) -> (x*y=w238:dbl)
              n94 = local read "Scan Continuously"() -> (w239:bool)
              n95 = call-poly <vilib>:"Number of Waveform Samples.vi"("waveform in"=w247) -> ("number of samples"=w246:i32)  [unwired: 8 in, 2 out]
              n96 = call-poly <vilib>:"DAQmx Timing.vi"("task/channels in"=w253, "samples per channel"=w246, "rate"=w238) -> ("task out"=w261:refnum<k21>, "error out"=w245:errorcluster)  [unwired: 11 in]
              n97 = call-poly <vilib>:"DAQmx Write.vi"("task/channels in"=w261, "data"=w249, "error in"=w245) -> ("task out"=w259:refnum<k21>, "error out"=w258:errorcluster)  [unwired: 10 in, 1 out]
              n98 = case shown="True" w239 {
                tunnel: w252 -> [w276 w284]
                tunnel: [w277 w283] -> _
                tunnel: w251 -> [w278 w282]
                frame False {
                  n99 = Bundle("Mode"=ModeEnum."Idle", "Microscope Settings"=w278) -> (w279:cluster{"Mode":T5, "Microscope Settings":T1})  [unwired: 1 in]
                  n100 = Enqueue Element(queue=w276, element=w279) -> (queue out=w277:refnum<queue>)  [unwired: 2 in, 2 out]
                }
                frame True {
                  n101 = Bundle("Mode"=ModeEnum."runWaves", "Microscope Settings"=w282) -> (w281:cluster{"Mode":T5, "Microscope Settings":T1})  [unwired: 1 in]
                  n102 = Enqueue Element(queue=w284, element=w281) -> (queue out=w283:refnum<queue>)  [unwired: 2 in, 2 out]
                }
              }
              n103 = disable-structure shown="Disabled" {
                disable-tunnel: _ -> [w272 _]
                disable-tunnel: w260 -> [w270 _]
                disable-tunnel: w258 -> [w267 w273]
                disable-tunnel: [w266 w273] -> w242
                disable-tunnel: [w264 w274] -> w256
                disable-tunnel: w254 -> [w262 w274]
                frame Disabled {
                  n104 = call-poly <vilib>:"DAQmx Timing.vi"("task/channels in"=w262, "rate"=w272) -> ("task out"=w271:refnum<k21>)  [unwired: 12 in, 1 out]
                  n105 = call-poly <vilib>:"DAQmx Write.vi"("task/channels in"=w271, "data"=w270) -> ("task out"=w269:refnum<k21>, "error out"=w268:errorcluster)  [unwired: 11 in, 1 out]
                  n106 = Merge Errors(w267, w268) -> (w266:errorcluster)
                  n107 = call <vilib>:"DAQmx Start Task.vi"("task/channels in"=w269, "error in"=w266) -> ("task out"=w265:refnum<k21>, "error out"=w263:errorcluster)  [unwired: 12 in]
                  n108 = call <vilib>:"DAQmx Wait Until Done.vi"("task/channels in"=w265, "error in"=w263) -> ("task out"=w264:refnum<k21>)  [unwired: 12 in, 1 out]
                }
                frame Enabled {
                }
              }
              n109 = call <vilib>:"DAQmx Start Task.vi"("task/channels in"=w259, "error in"=w242) -> ("task out"=w257:refnum<k21>, "error out"=w255:errorcluster)  [unwired: 12 in]
              n110 = call <vilib>:"DAQmx Wait Until Done.vi"("task/channels in"=w257, "error in"=w255) -> ("task out"=w244:refnum<k21>)  [unwired: 12 in, 1 out]
              n111 = call <vilib>:"DAQmx Stop Task.vi"("task/channels in"=w244, "error in"=w242) -> ("task out"=w243:refnum<k21>)  [unwired: 12 in, 1 out]
            }
            frame "stop" {
            }
          }
        }
        n112 = while {
          tunnel: w169 -> [w434]
          shift-right: [w433] -> _
          shift-left: _ -> [w432]
          tunnel: w161 -> [w430]
          stop <- w435 stop-if-true
          n113 = event shown="[1] \"Microscope Settings\": Value Change" {
            selector: _ -> [_ _ _ _]
            dyn-events: _ -> [_ _ _ _]
            timeout: 10 -> [_ _ _ _]
            tunnel: [w436 _ _ _] -> w435
            tunnel: w434 -> [_ w441 _ _]
            tunnel: [_ w438 _ w482] -> w433
            tunnel: w432 -> [_ _ w479 _]
            tunnel: [_ _ w478 _] -> _
            tunnel: w430 -> [_ w437 w477 _]
            event "stop": Value Change {
              n114 = event-data() -> ()  [unwired: 1 in, 6 out]
              n115 = local read "stop"() -> (w436:bool)
            }
            event Value Change {
              # "Live video for Calibration and 2D\nScan Modes.\n\nIdle Video for MultiD Scan modes\nUNTIL Begin Scan Button pressed?\n\nMultiD is waiting for trigger"
              n116 = event-data() -> ("NewVal"=w440:T1)  [unwired: 1 in, 5 out]
              n117 = Unbundle By Name(w440) -> ("Mode"=w439:enum16{"X", "XY", "XYZ", "XYZT", "XYZC"})
              n118 = case shown="\"XYZ\"" w439 {
                tunnel: w441 -> [w452 w464 w473 _ _]
                tunnel: w440 -> [w444 w456 w467 w475 w476]
                tunnel: [w444 w456 w467 w475 w476] -> w438
                tunnel: w437 -> [w443 w455 _ _ _]
                frame "X" {
                  w446 = ModeEnum."generateWaves"  # Mode
                  w447 = 0 ("timeout in ms (-1)")
                  w442 = 1.0 items=["Internal"=1.0, "External"=2.0] ("Trigger Source")
                  n119 = property on="Trigger Source" class="Ring (strict)"("Value"=w442) -> ()  [unwired: 2 in, 2 out]
                  n120 = Bundle("Enum"=CameraControlTypeDef."Readout Mode", "Trigger Source"=w442, "timeout in ms (-1)"=w447) -> (w451:T15)  [unwired: 1 in]
                  n121 = Enqueue Element(queue=w452, element=w451) -> (queue out=w449:refnum<queue>)  [unwired: 2 in, 2 out]
                  n122 = Bundle("Enum"=CameraControlTypeDef."Preview", "Trigger Source"=w442, "timeout in ms (-1)"=w447) -> (w450:T15)  [unwired: 1 in]
                  n123 = Bundle("Mode"=w446, "NewVal"=w444) -> (w445:cluster{"Mode":T5, "NewVal":T1})  [unwired: 1 in]
                  n124 = Enqueue Element(queue=w449, element=w450) -> ()  [unwired: 2 in, 3 out]
                  n125 = Enqueue Element(queue=w443, element=w445) -> ()  [unwired: 2 in, 3 out]
                }
                frame "XY" {
                  w458 = ModeEnum."generateWaves"  # Mode
                  w459 = 0 ("timeout in ms (-1)")
                  w454 = 2.0 items=["Internal"=1.0, "External"=2.0] ("Trigger Source")
                  n126 = property on="Trigger Source" class="Ring (strict)"("Value"=w454) -> ()  [unwired: 2 in, 2 out]
                  n127 = Bundle("Enum"=CameraControlTypeDef."Readout Mode", "Trigger Source"=w454, "timeout in ms (-1)"=w459) -> (w463:T15)  [unwired: 1 in]
                  n128 = Enqueue Element(queue=w464, element=w463) -> (queue out=w460:refnum<queue>)  [unwired: 2 in, 2 out]
                  n129 = Bundle("Mode"=w458, "NewVal"=w456) -> (w457:cluster{"Mode":T5, "NewVal":T1})  [unwired: 1 in]
                  n130 = Bundle("Enum"=CameraControlTypeDef."Preview", "Trigger Source"=w454, "timeout in ms (-1)"=w459) -> (w462:T15)  [unwired: 1 in]
                  n131 = Enqueue Element(queue=w455, element=w457) -> ()  [unwired: 2 in, 3 out]
                  n132 = Enqueue Element(queue=w460, element=w462) -> ()  [unwired: 2 in, 3 out]
                  n133 = property on="Microscope Settings" class="Clust (strict)" props=["Value"]() -> ()  [unwired: 2 in, 3 out]
                }
                frame "XYZ" {
                  w468 = 0 ("timeout in ms (-1)")
                  w466 = 2.0 items=["Internal"=1.0, "External"=2.0] ("Trigger Source")
                  n134 = property on="Trigger Source" class="Ring (strict)"("Value"=w466) -> ()  [unwired: 2 in, 2 out]
                  n135 = Bundle("Enum"=CameraControlTypeDef."Readout Mode", "Trigger Source"=w466, "timeout in ms (-1)"=w468) -> (w472:T15)  [unwired: 1 in]
                  n136 = Enqueue Element(queue=w473, element=w472) -> (queue out=w471:refnum<queue>)  [unwired: 2 in, 2 out]
                  n137 = Bundle("Enum"=CameraControlTypeDef."Idle", "Trigger Source"=w466, "timeout in ms (-1)"=w468) -> (w470:T15)  [unwired: 1 in]
                  n138 = Enqueue Element(queue=w471, element=w470) -> ()  [unwired: 2 in, 3 out]
                }
                frame "XYZT" {
                }
                frame "XYZC" {
                }
              }
            }
            event "Scan": Value Change {
              w481 = ModeEnum."runWaves"  # Mode
              n139 = event-data() -> ()  [unwired: 1 in, 6 out]
              n140 = Bundle("Mode"=w481, "Value"=w479) -> (w480:cluster{"Mode":T5, "Value":T1})  [unwired: 1 in]
              n141 = Enqueue Element(queue=w477, element=w480) -> (queue out=w478:refnum<queue>)  [unwired: 2 in, 2 out]
            }
            event Timeout {
              n142 = event-data() -> ()  [unwired: 1 in, 3 out]
              n143 = property on="Microscope Settings" class="Clust (strict)"() -> ("Value"=w482:T1)  [unwired: 2 in, 2 out]
            }
          }
        }
        n144 = Merge Errors(w180, w181) -> (w182:errorcluster)
      }
      frame "deinit" {
        n145 = call <vilib>:"DAQmx Stop Task.vi"("task/channels in"=w493) -> ("task out"=w494:refnum<k21>)  [unwired: 13 in, 1 out]
        n146 = call <vilib>:"DAQmx Stop Task.vi"("task/channels in"=w495) -> ("task out"=w496:refnum<k21>)  [unwired: 13 in, 1 out]
        n147 = call <vilib>:"DAQmx Clear Task.vi"("task in"=w494) -> ("error out"=w490:errorcluster)  [unwired: 14 in]
        n148 = call "tm_stopcapture.vi"("error in (no error)"=w505, "Handle in"=w501) -> ("error out"=w508:errorcluster, "Handle out"=w507:u32)  [unwired: 8 in]
        n149 = call <vilib>:"DAQmx Clear Task.vi"("task in"=w496) -> ("error out"=w491:errorcluster)  [unwired: 14 in]
        n150 = call "tm_unpreparecapture.vi"("error in (no error)"=w508, "Handle in"=w507) -> ("error out"=w509:errorcluster, "Handle out"=w506:u32)  [unwired: 8 in]
        n151 = call "tm_closecamera.vi"("error in (no error)"=w509, "Handle in"=w506) -> ("error out"=w510:errorcluster)  [unwired: 9 in]
        n152 = Flush Queue(queue=w483) -> (queue out=w489:refnum<queue>)  [unwired: 1 in, 2 out]
        n153 = call "tm_deinitialize.vi"("error in (no error)"=w510) -> ("error out"=w486:errorcluster)  [unwired: 10 in]
        n154 = Release Queue(queue=w484, error in (no error)=w486) -> (error out=w503:errorcluster)  [unwired: 1 in, 2 out]
        n155 = Release Queue(queue=w489) -> (error out=w492:errorcluster)  [unwired: 2 in, 2 out]
        n156 = Flush Queue(queue=w488, error in (no error)=w486) -> (queue out=w487:refnum<queue>, error out=w485:errorcluster)  [unwired: 1 out]
        n157 = Release Queue(queue=w487, error in (no error)=w485) -> (error out=w502:errorcluster)  [unwired: 1 in, 2 out]
        n158 = Merge Errors(w503, w502, w492, w491, w490) -> (w504:errorcluster)
      }
    }
    n159 = Or(x="stop", y=w22) -> (x .or. y?=w23:bool)
  }
  "error IO" <- w10
  n160 = disable-structure shown="Enabled" {
    frame Disabled {
      # "Parallise decode buffer"
      n161 = call "tm_startcapture_b.vi"() -> ()  [unwired: 10 in, 2 out]
      n162 = call "tm_waitnextframe.vi"() -> ()  [unwired: 8 in, 4 out]
      n163 = call "tm_getframe_a.vi"() -> ()  [unwired: 7 in, 5 out]
    }
    frame Enabled {
    }
  }
